vi "D Set Power Range.vi"(7 "Source Power(Off:F)":bool, 8 "error in (no error)":errorcluster, 9 "Power Range Mode(Manual:F)":bool, 10 "Manual Power Range (1)":u32(ring)=1 items=["0", "1", "2", "3", "4", "5", "6", "7"], 11 "VISA resource name":refnum<visa-resource-name>) -> (0 "error out":errorcluster, 3 "VISA resource name out":refnum<visa-resource-name>)   [LabVIEW 2018, in "Agilent 87XX Series.lvlib"]
doc: "This vi sets the power range. Only works on the HP 8753D."
uses:
  Agilent 87XX Series.lvlib
panel:
  # "Auto"
  # "Manual"
  # "On"
  # "Off"
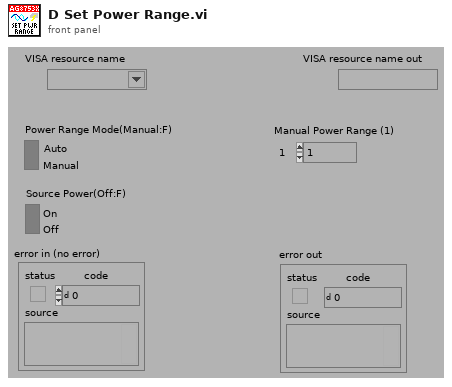
[diagram p1: front panel]
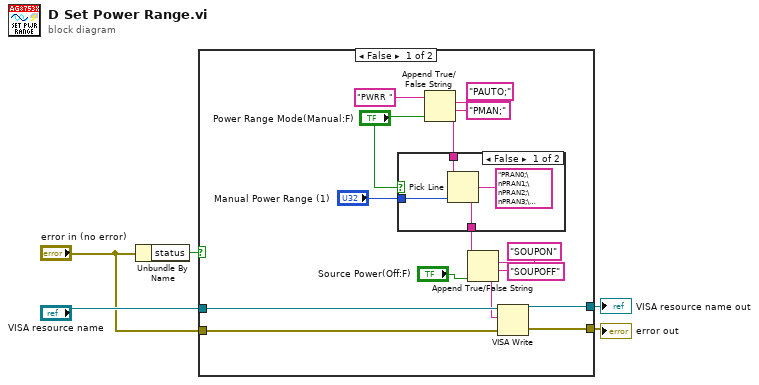
[diagram p0: block diagram]
diagram:
  n1 = Unbundle By Name("error in (no error)") -> ("status"=w5:bool)
  n2 = case shown="False" w5 {
    tunnel: "VISA resource name" -> [w16 w27]
    tunnel: "error in (no error)" -> [w15 w26]
    tunnel: [w14 w26] -> w2
    tunnel: [w13 w27] -> w1
    frame False {
      n3 = Append True/False String(1:"Power Range Mode(Manual:F)", 2:"PMAN;", 3:"PAUTO;", 4:"PWRR ") -> (0:w7:string)
      n4 = case shown="False" "Power Range Mode(Manual:F)" {
        tunnel: [w24 w25] -> w12
        tunnel: w7 -> [w22 w25]
        tunnel: "Manual Power Range (1)" -> [w21 _]
        frame False {
          n5 = Pick Line(string ("")=w22, multi-line string="PRAN0;\nPRAN1;\nPRAN2;\nPRAN3;\nPRAN4;\nPRAN5;\nPRAN6;\nPRAN7;", line index=w21) -> (output string=w24:string)
        }
        frame True {
        }
      }
      n6 = Append True/False String(1:"Source Power(Off:F)", 2:"SOUPOFF", 3:"SOUPON", 4:w12) -> (0:w10:string)
      n7 = VISA Write(VISA resource name=w16, write buffer=w10, error in (no error)=w15) -> (VISA resource name out=w13:refnum<visa-resource-name>, error out=w14:errorcluster)  [unwired: 1 out]
    }
    frame True {
    }
  }
  "VISA resource name out" <- w1
  "error out" <- w2
